vi "Windows Title - Copy.vi"(8 "error in (no error)":errorcluster, 10 "Windows Title Value":string, 11 "CallActorCenter in":refnum<class "CallActorCenter.lvclass">) -> (0 "error out":errorcluster, 3 "CallActorCenter out":refnum<class "CallActorCenter.lvclass">)   [LabVIEW 2021]
uses:
  CallActorCenter.lvclass
  C:/Program Files (x86)/National Instruments/LabVIEW 2021/vi.lib/ActorFramework/Actor/Actor.lvclass
  <vilib>/ActorFramework/Actor/Actor.lvclass/Actor.ctl
  Source_Public/Public Interface/Windows Title Messages/Windows Title Msg/Windows Title Msg.lvclass/Windows Title Msg.ctl
  <vilib>/ActorFramework/Message Enqueuer/Message Enqueuer.lvclass/Message Enqueuer.ctl
  <vilib>/ActorFramework/Message Enqueuer/Enqueue.vi
  Source_Public/Public Interface/Windows Title Messages/Windows Title Msg/Windows Title Msg.lvclass
  C:/Program Files (x86)/National Instruments/LabVIEW 2021/vi.lib/ActorFramework/Message/Message.lvclass
  <vilib>/ActorFramework/Message Priority Queue/Priority Enqueue.vi
  <vilib>/ActorFramework/Actor/Actor.lvclass
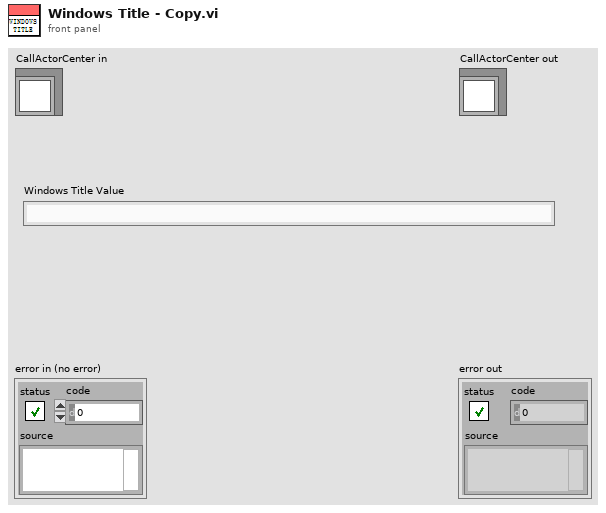
[diagram p1: front panel]
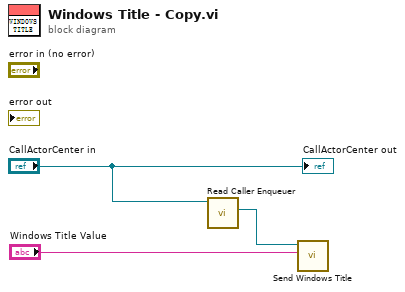
[diagram p0: block diagram]
diagram:
  n1 = call <vilib>:"Read Caller Enqueuer.vi"("Actor"="CallActorCenter in") -> ("Caller Enqueuer"=w2:refnum<class "Message Enqueuer.lvclass">)  [unwired: 10 in]
  n2 = call "Send Windows Title.vi"("Windows Title Value"="Windows Title Value", "Message Enqueuer"=w2) -> ()  [unwired: 8 in, 2 out]
  "CallActorCenter out" <- "CallActorCenter in"
